vi "GenerateDisplayData.vi"(7 "Index":i32, 8 "Error In":errorcluster, 10 "UI Controls Refnum":T1, 11 "2D Data IN":string[][](array[string])) -> (0 "Error Out":errorcluster, 1 "Notes":string[][](array[string]), 2 "Big Table":string[][](array[string]), 3 "Plot Data OUT":cluster{dbl[], dbl[]}[](array[cluster]))   [LabVIEW 2012]
doc: "Thsi VI takes the Position data (2D string array) and generates the data to populate:\n1. Big table\n2. Notes Table\n4. XY Graph\n5. Saved Image"
uses:
  Custom Control and Typedefs/UI Controls Refnum.ctl
  Custom Control and Typedefs/ChannelSelector_for_PosSave.ctl
  Custom Controls/PositionSaveMod.ctl
  Custom Control and Typedefs/Overlay Control.ctl
panel:
  # "Red (Current Image)"
  # "Green (Saved Image)"
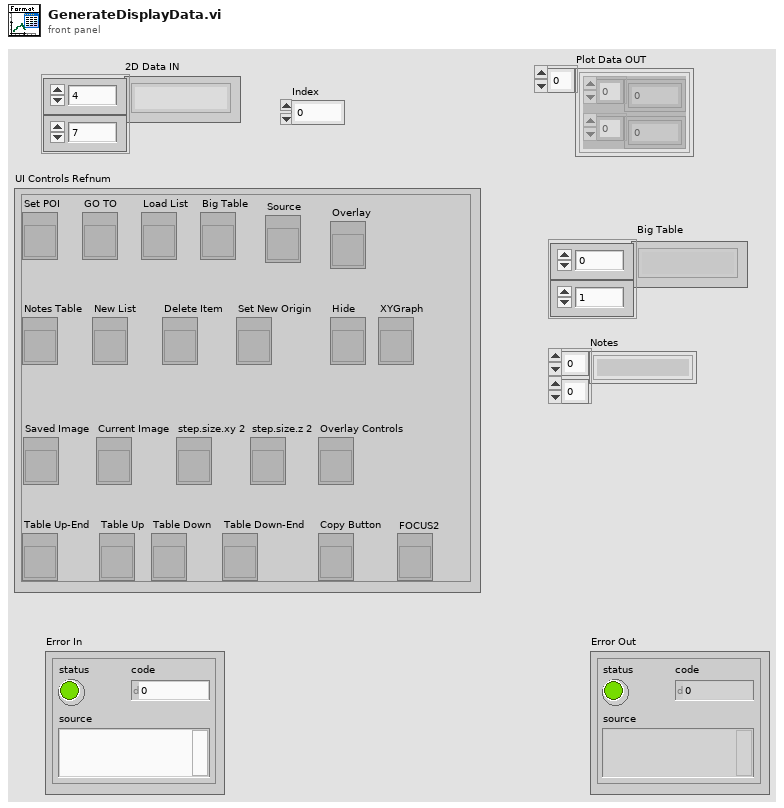
[diagram p1: front panel]
types:
  T1 = typedef "UI Controls Refnum.ctl" = cluster{"GO TO":refnum<vi>, "Load List":refnum<vi>, "Big Table":refnum<vi>, "Notes Table":refnum<vi>, "New List":refnum<vi>, "Delete Item":refnum<vi>, "Set New Origin":refnum<vi>, "Set POI":refnum<vi>, "Saved Image":refnum<vi>, "Current Image":refnum<vi>, "step.size.xy 2":refnum<vi>, "step.size.z 2":refnum<vi>, "Source":refnum<vi>, "Table Up-End":refnum<vi>, "Table Up":refnum<vi>, "Table Down":refnum<vi>, "Table Down-End":refnum<vi>, "Copy Button":refnum<vi>, "Hide":refnum<vi>, "Overlay Controls":refnum<vi>, "Overlay":refnum<vi>, "XYGraph":refnum<vi>, "FOCUS2":refnum<vi>}
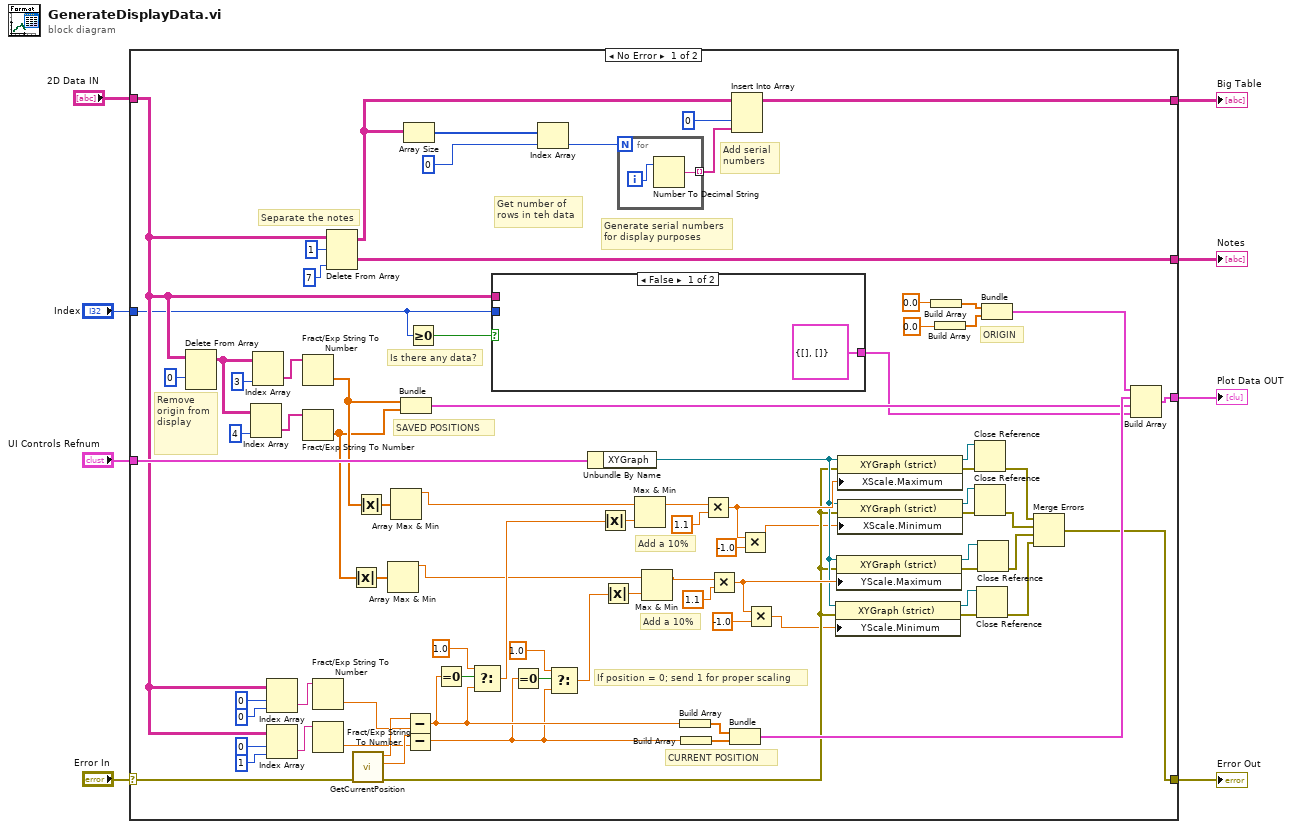
[diagram p0: block diagram]
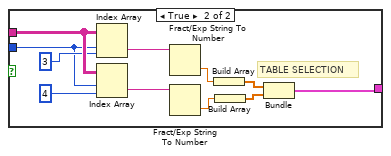
[diagram p2: hidden frame]
diagram:
  n1 = case shown="No Error" "Error In" {
    selector: "Error In" -> [w77 w107]
    tunnel: "2D Data IN" -> [w12 w106]
    tunnel: [w86 w106] -> w6
    tunnel: [w43 w107] -> w5
    tunnel: [w82 w106] -> w4
    tunnel: [w64 _] -> w3
    tunnel: "UI Controls Refnum" -> [w54 _]
    tunnel: "Index" -> [w10 _]
    frame No Error {
      # "Is there any data?"
      # "SAVED POSITIONS"
      # "If position = 0; send 1 for proper scaling"
      # "Add a 10%"
      # "Add a 10%"
      # "Remove origin from \ndisplay"
      # "ORIGIN"
      # "CURRENT POSITION"
      # "Separate the notes"
      # "Add serial \nnumbers"
      # "Generate serial numbers\nfor display purposes"
      # "Get number of\nrows in teh data"
      n2 = Delete From Array(array=w12, index (row)=0) -> (array with subset deleted=w55:string[][])  [unwired: 2 in, 1 out]
      n3 = Index Array(array=w55, index (col)=4 ("disabled index (col)")) -> (element=w80:string[])  [unwired: 1 in]
      n4 = Index Array(array=w55, index (col)=3 ("disabled index (col)")) -> (element=w79:string[])  [unwired: 1 in]
      n5 = Index Array(array=w12, index (row)=0, index (col)=0 ("disabled index (col)")) -> (element=w72:string)
      n6 = Index Array(array=w12, index (row)=0, index (col)=1 ("disabled index (col)")) -> (element=w71:string)
      n7 = Fract/Exp String To Number(string=w79) -> (number=w18:dbl[])  [unwired: 3 in, 1 out]
      n8 = Fract/Exp String To Number(string=w80) -> (number=w15:dbl[])  [unwired: 3 in, 1 out]
      n9 = Fract/Exp String To Number(string=w72) -> (number=w68:dbl)  [unwired: 3 in, 1 out]
      n10 = Fract/Exp String To Number(string=w71) -> (number=w67:dbl)  [unwired: 3 in, 1 out]
      n11 = Delete From Array(array=w12, length=1, index (col)=7 ("disabled index (col)")) -> (deleted portion=w82:string[][], array with subset deleted=w84:string[][])  [unwired: 1 in]
      n12 = Absolute Value(x=w15) -> (abs(x)=w14:dbl[])
      n13 = call "GetCurrentPosition.vi"("Error In"=w77) -> ("Error Out"=w35:errorcluster, "Y"=w69:dbl, "X"=w70:dbl)  [unwired: 7 in, 1 out]
      n14 = Absolute Value(x=w18) -> (abs(x)=w17:dbl[])
      n15 = Array Max & Min(array=w14) -> (max value=w13:dbl)  [unwired: 3 out]
      n16 = Array Max & Min(array=w17) -> (max value=w16:dbl)  [unwired: 3 out]
      n17 = Bundle(w18, w15) -> (w62:cluster{dbl[], dbl[]})  [unwired: 1 in]
      n18 = Array Size(array=w84) -> (size(s)=w87:i32[])
      n19 = Subtract(x=w70, y=w68) -> (x-y=w24:dbl)
      n20 = Subtract(x=w69, y=w67) -> (x-y=w20:dbl)
      n21 = Greater Or Equal To 0?(x=w10) -> (x >= 0?=w9:bool)
      n22 = Equal To 0?(x=w24) -> (x = 0?=w26:bool)
      n23 = Select(t=1.0, s=w26, f=w24) -> (s? t:f=w23:dbl)
      n24 = case shown="False" w9 {
        tunnel: w12 -> [_ w103]
        tunnel: w10 -> [_ w100]
        tunnel: [cluster{dbl[], dbl[]} {[], []} w93] -> w11
        frame False {
        }
        frame True {
          # "TABLE SELECTION"
          n25 = Index Array(array=w103, index (row)=w100, index (col)=3 ("index (row)")) -> (element=w99:string)
          n26 = Index Array(array=w103, index (row)=w100, index (col)=4 ("index (row)")) -> (element=w98:string)
          n27 = Fract/Exp String To Number(string=w99) -> (number=w96:dbl)  [unwired: 3 in, 1 out]
          n28 = Fract/Exp String To Number(string=w98) -> (number=w97:dbl)  [unwired: 3 in, 1 out]
          n29 = Build Array(w96) -> (w95:dbl[])
          n30 = Build Array(w97) -> (w94:dbl[])
          n31 = Bundle(w95, w94) -> (w93:cluster{dbl[], dbl[]})  [unwired: 1 in]
        }
      }
      n32 = Equal To 0?(x=w20) -> (x = 0?=w21:bool)
      n33 = Index Array(array=w87, index=0) -> (element=w89:i32)
      n34 = Select(t=1.0, s=w21, f=w20) -> (s? t:f=w19:dbl)
      n35 = Unbundle By Name(w54) -> ("XYGraph"=w36:refnum<vi>)
      n36 = Absolute Value(x=w23) -> (abs(x)=w30:dbl)
      n37 = Absolute Value(x=w19) -> (abs(x)=w29:dbl)
      n38 = for {
        N: w89 -> [_]
        tunnel: [w104] -> w91 mode=indexing
        i -> [w105]
        n39 = Number To Decimal String(number=w105) -> (decimal integer string=w104:string)  [unwired: 1 in]
      }
      n40 = Max & Min(x=w16, y=w30) -> (max(x,y)=w53:dbl)  [unwired: 1 out]
      n41 = Max & Min(x=w13, y=w29) -> (max(x,y)=w48:dbl)  [unwired: 1 out]
      n42 = Build Array(w24) -> (w66:dbl[])
      n43 = Build Array(w20) -> (w65:dbl[])
      n44 = Multiply(x=w53, y=1.1) -> (x*y=w40:dbl)
      n45 = Multiply(x=w48, y=1.1) -> (x*y=w37:dbl)
      n46 = Bundle(w66, w65) -> (w63:cluster{dbl[], dbl[]})  [unwired: 1 in]
      n47 = Insert Into Array(array=w84, index (col)=0 ("disabled index (col)"), new element=w91) -> (w86:string[][])  [unwired: 1 in]
      n48 = Multiply(x=w40, y=-1.0) -> (x*y=w28:dbl)
      n49 = Multiply(x=w37, y=-1.0) -> (x*y=w27:dbl)
      n50 = property class="XYGraph (strict)"(reference=w36, error in=w35, "YScale.Minimum"=w27) -> (reference out=w39:refnum<vi>, error out=w38:errorcluster)
      n51 = property class="XYGraph (strict)"(reference=w36, error in=w35, "YScale.Maximum"=w37) -> (reference out=w44:refnum<vi>, error out=w45:errorcluster)
      n52 = property class="XYGraph (strict)"(reference=w36, error in=w35, "XScale.Maximum"=w40) -> (reference out=w46:refnum<vi>, error out=w47:errorcluster)
      n53 = property class="XYGraph (strict)"(reference=w36, error in=w35, "XScale.Minimum"=w28) -> (reference out=w42:refnum<vi>, error out=w41:errorcluster)
      n54 = Build Array(0.0 ("number")) -> (w59:dbl[])
      n55 = Build Array(0.0 ("number")) -> (w58:dbl[])
      n56 = Close Reference(reference=w46, error in (no error)=w47) -> (error out=w34:errorcluster)
      n57 = Close Reference(reference=w42, error in (no error)=w41) -> (error out=w33:errorcluster)
      n58 = Close Reference(reference=w39, error in (no error)=w38) -> (error out=w31:errorcluster)
      n59 = Close Reference(reference=w44, error in (no error)=w45) -> (error out=w32:errorcluster)
      n60 = Bundle(w59, w58) -> (w57:cluster{dbl[], dbl[]})  [unwired: 1 in]
      n61 = Merge Errors(w34, w33, w32, w31) -> (w43:errorcluster)
      n62 = Build Array(w57, w63, w62, w11) -> (w64:cluster{dbl[], dbl[]}[])
    }
    frame Error {
    }
  }
  "Error Out" <- w5
  "Big Table" <- w6
  "Notes" <- w4
  "Plot Data OUT" <- w3
